vi "Request New Port ID.vi"(8 "error in":errorcluster, 10 "Assert ID":string, 11 "Service Action Base in":refnum<class "Service Action Base.lvclass">) -> (0 "error out":errorcluster, 2 "Create New Link":bool, 3 "Service Action Base out":refnum<class "Service Action Base.lvclass">, 4 "New Port Number":u16)   [LabVIEW 2016, in "Assert API Components.lvlib" / "Assert Service.lvlib" / "Service Action Base.lvclass"]
doc: "Requests a new port ID to be used to open up UDP comms on. Increments the port count so the next request gets a different port number"
uses:
  Service Action Base.lvclass
  Service Action Base.lvclass/Service Action Base.ctl
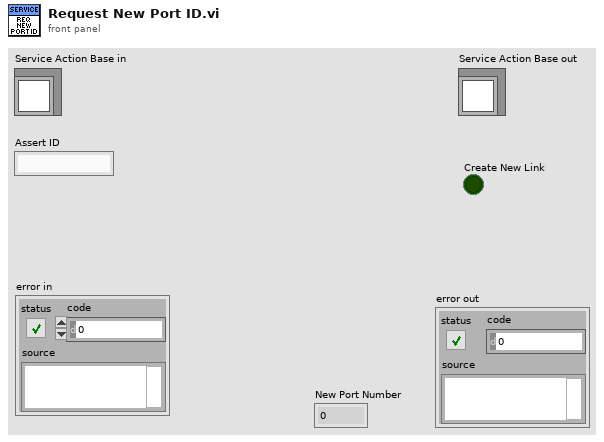
[diagram p1: front panel]
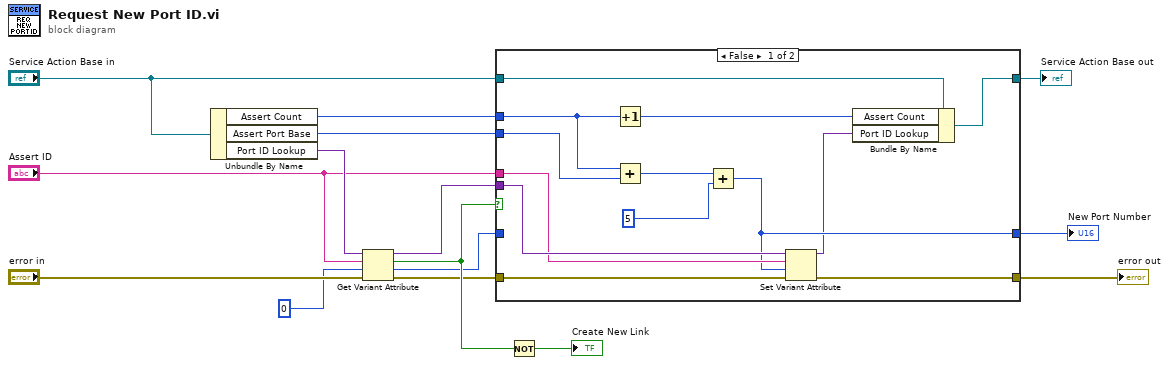
[diagram p0: block diagram]
diagram:
  n1 = Unbundle By Name("Service Action Base in") -> ("Assert Count"=w3:u16, "Assert Port Base"=w2:u16, "Port ID Lookup"=w12:variant)
  n2 = Get Variant Attribute(Variant=w12, name="Assert ID", default value (empty Variant)=u16 0 ("y"), error in="error in") -> (duplicate Variant=w9:variant, found=w10:bool, value=w4:u16, error out=w8:errorcluster)
  n3 = case shown="False" w10 {
    tunnel: "Service Action Base in" -> [w28 w31]
    tunnel: w2 -> [w27 _]
    tunnel: w3 -> [w24 _]
    tunnel: [w23 w31] -> w14
    tunnel: [w18 w30] -> w13
    tunnel: w9 -> [w21 _]
    tunnel: w8 -> [w20 w29]
    tunnel: "Assert ID" -> [w19 _]
    tunnel: [w17 w29] -> w6
    tunnel: w4 -> [_ w30]
    frame False {
      n4 = Increment(x=w24) -> (x+1=w22:u16)
      n5 = Add(x=w24, y=w27) -> (x+y=w26:u16)
      n6 = Add(x=w26, y=u16 5) -> (x+y=w18:u16)
      n7 = Set Variant Attribute(Variant=w21, name=w19, value=w18, error in=w20) -> (Variant out=w16:variant, error out=w17:errorcluster)  [unwired: 1 out]
      n8 = Bundle By Name(cluster=w28, "Assert Count"=w22, "Port ID Lookup"=w16) -> (w23:refnum<class "Service Action Base.lvclass">)
    }
    frame True {
    }
  }
  "Service Action Base out" <- w14
  "New Port Number" <- w13
  "error out" <- w6
  n9 = Not(x=w10) -> (.not. x?=→"Create New Link":bool)
